vi "Core-CatchAndClearError.vi"(6 "error in (no error)":errorcluster caption="错误输入（无错误）", 9 "ErrorQ":refnum<queue>) -> (0 "error out":errorcluster caption="错误输出")   [LabVIEW 2014]
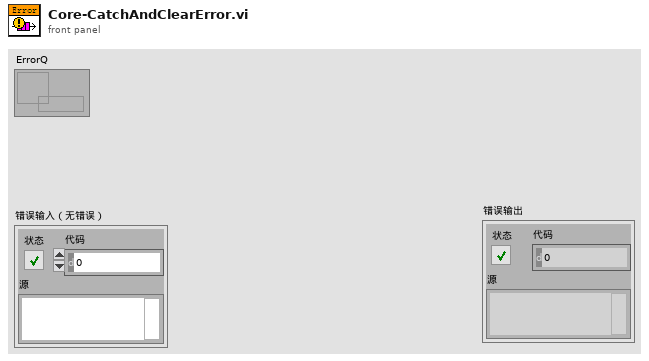
[diagram p1: front panel]
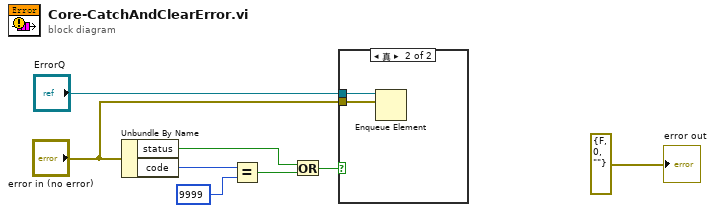
[diagram p0: block diagram]
diagram:
  n1 = Unbundle By Name("error in (no error)") -> ("status"=w7:bool, "code"=w5:i32)
  n2 = Equal?(x=w5, y=9999) -> (x = y?=w8:bool)
  n3 = Or(x=w7, y=w8) -> (x .or. y?=w6:bool)
  n4 = case shown="真" w6 {
    tunnel: "error in (no error)" -> [_ w10]
    tunnel: "ErrorQ" -> [_ w9]
    frame False {
    }
    frame True {
      n5 = Enqueue Element(queue=w9, element=w10) -> ()  [unwired: 2 in, 3 out]
    }
  }
  "error out" <- errorcluster {"status"=FALSE, "code"=0, "source"=""} ("错误常量")
